vi "get all tags in collection.vi"(11 "tag collection in":refnum<class "tag collection.lvclass">) -> (2 "tags":refnum<class "tag descriptor.lvclass">[](array[class]), 3 "tag collection out":refnum<class "tag collection.lvclass">)   [LabVIEW 2013, in "tag bus.lvlib" / "tag collection.lvclass"]
uses:
  tag collection.lvclass
  tag/tag descriptor.lvclass
  tag collection.lvclass/tag collection.ctl
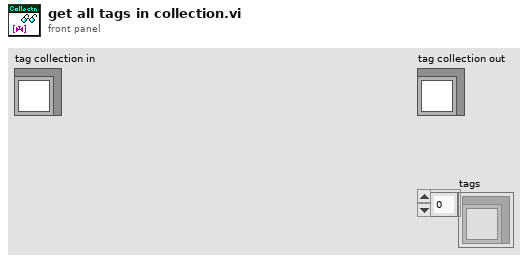
[diagram p1: front panel]
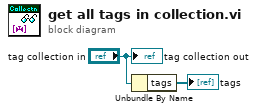
[diagram p0: block diagram]
diagram:
  n1 = Unbundle By Name("tag collection in") -> ("tags"=→"tags":refnum<class "tag descriptor.lvclass">[])
  "tag collection out" <- "tag collection in"
